vi "Read Proxy Enq.vi"(11 "Target in":refnum<class "Target.lvclass">) -> (2 "Actor Framework:Message Enqueuer":refnum<class "Message Enqueuer.lvclass">, 3 "Target out":refnum<class "Target.lvclass">)   [LabVIEW 2014, in "Target.lvlib" / "Target.lvclass"]
uses:
  Target.lvclass
  <vilib>/ActorFramework/Message Enqueuer/Message Enqueuer.lvclass
  Target.lvclass/Target.ctl
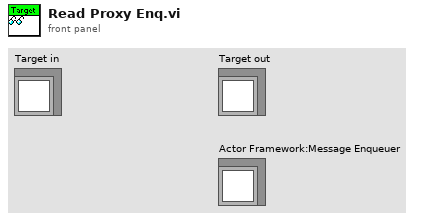
[diagram p1: front panel]
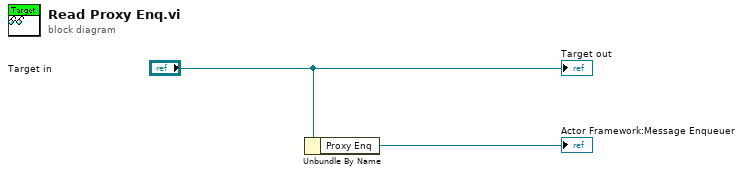
[diagram p0: block diagram]
diagram:
  n1 = Unbundle By Name("Target in") -> ("Proxy Enq"=→"Actor Framework:Message Enqueuer":refnum<class "Message Enqueuer.lvclass">)
  "Target out" <- "Target in"
